vi "Link Channel.vi"(8 "error in (no error)":errorcluster, 11 "CIF_UI in":refnum<class "CIF_UI.lvclass">) -> (0 "error out":errorcluster, 3 "CIF_UI out":refnum<class "CIF_UI.lvclass">)   [LabVIEW 2021, in "CIF_UI.lvclass"]
uses:
  CIF_UI.lvclass
  CIF_UI.lvclass/CIF_UI.ctl
  CIFCore/Grpc/CIFCoreWrapper/CIFCoreWrapper.lvlib
  CIFCore/Grpc/CIFCoreChannel_client/RPC Messages/cif_channelcore_ConnectSubscriber.ctl
  CIFCore/Grpc/CIFCoreChannel_client/CIFCoreChannel_client.lvlib
  CIFCore/Common/CIFCoreCommon.lvlib
  CIFCore/Common/Typedef/Errors.ctl
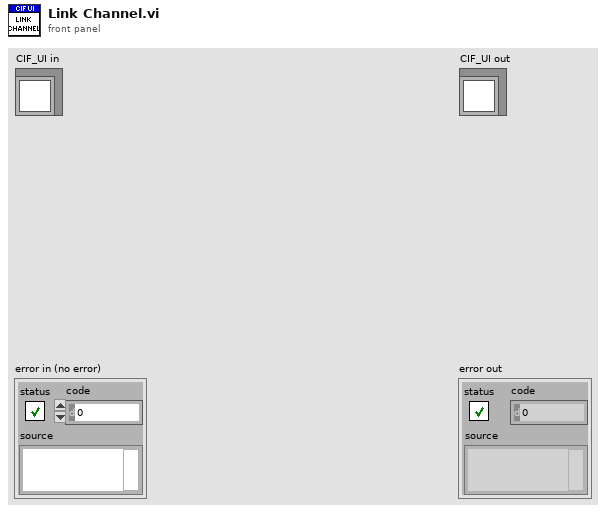
[diagram p1: front panel]
types:
  T1 = typedef "CIF_UI.lvclass/Plugin Connection Map.ctl" = map{string, T2}
  T2 = typedef "CIF_UI.lvclass/Plugin Connections.ctl" = cluster{"gRPC ID":T3, "Plugin info":T4}
  T3 = typedef "grpc-lvsupport-release.lvlib/grpcId.ctl" = u64
  T4 = typedef "CIF_Manager_client.lvlib/cif_manager_PluginInfo.ctl" = cluster{"plugin_name":string, "plugin_type":string, "grpc_port":i32, "plugin_version":T5, "status":T6}
  T5 = typedef "CIF_Manager_client.lvlib/cif_manager_PluginVersion.ctl" = cluster{"major_version":i32, "minor_version":i32, "fix_version":i32, "build_version":i32}
  T6 = typedef "CIF_Manager_client.lvlib/cif_plugincore_StatusData.ctl" = cluster{"state":T7, "timing_statistics":T8, "fifo_statistics":T10, "error":T11, "monitor_doubles":T12, "monitor_u64s":T13, "monitor_i64s":T14}
  T7 = typedef "CIF_Manager_client.lvlib/cif_plugincore_StatusData_State.ctl" = enum32{"NULL", "CREATING", "LISTENING", "RUNNING", "CLEANINGUP", "DESTROYING"}
  T8 = typedef "CIF_Manager_client.lvlib/cif_plugincore_TimingStatistics.ctl" = cluster{"period":T9, "wake_error":T9, "execute":T9, "housekeep":T9, "idle":T9}
  T9 = typedef "CIF_Manager_client.lvlib/cif_plugincore_TimingStatsBasic.ctl" = cluster{"max":i32, "min":i32}
  T10 = typedef "CIF_Manager_client.lvlib/cif_plugincore_FifoStatistics.ctl" = cluster{"from_t0":T9, "from_previous_plugin":T9, "output_error":T9}
  T11 = typedef "CIF_Manager_client.lvlib/cif_plugincore_Error.ctl" = cluster{"status":bool, "code":i32}
  T12 = typedef "CIF_Manager_client.lvlib/cif_plugincore_MonitorDoubles.ctl" = cluster{"double_1":dbl, "double_2":dbl, "double_3":dbl, "double_4":dbl}
  T13 = typedef "CIF_Manager_client.lvlib/cif_plugincore_MonitorU64.ctl" = cluster{"u64_1":u64, "u64_2":u64, "u64_3":u64, "u64_4":u64}
  T14 = typedef "CIF_Manager_client.lvlib/cif_plugincore_MonitorI64.ctl" = cluster{"i64_1":i64, "i64_2":i64, "i64_3":i64, "i64_4":i64}
  T15 = typedef "CIFCoreChannel_client.lvlib/cif_channelcore_ConnectSubscriber.ctl" = cluster{"subscriber_name":string, "publisher_name":string, "custom_connect":u8[]}
  T16 = typedef "CIFCoreCommon.lvlib/Errors.ctl" = enum16{"Invalid Clock ID", "Long Sleep", "gRPC Server Not Found", "Config Parse", "Timestamp Wrap", "Delayed Execution", "Duplicate Channel", "Missing Channel", "Incorrect Type", "Flatten Error", "Unflatten Data", "Unique Name", "Plugin Not Found", "Plugin Type Not Found", "Plugin Version Not Found", "Manager Not Found", "Numerical Issue", "Time Jump", "Clock ID Match", "Channel Length", "Plugin Connection"}
  T17 = typedef "CIF_UI.lvclass/Channel Connection.ctl" = cluster{"Subscriber Name":string, "Publisher Name":string, "Custom Data":string}
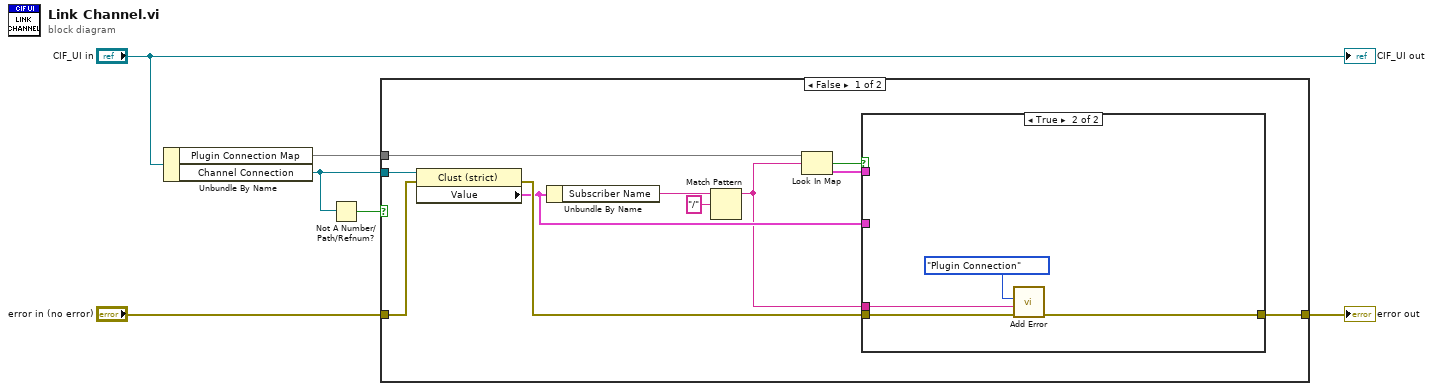
[diagram p0: block diagram]
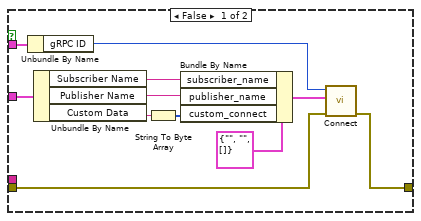
[diagram p2: hidden frame]
diagram:
  n1 = Unbundle By Name("CIF_UI in") -> ("Plugin Connection Map"=w4:T1, "Channel Connection"=w2:refnum<vi>)
  n2 = Not A Number/Path/Refnum?(number/path/refnum=w2) -> (NaN/Path/Refnum?=w1:bool)
  n3 = case shown="False" w1 {
    tunnel: "error in (no error)" -> [w17 w33]
    tunnel: w4 -> [w12 _]
    tunnel: [w9 w33] -> w3
    tunnel: w2 -> [w8 _]
    frame False {
      n4 = property class="Clust (strict)"(reference=w8, error in=w17) -> (error out=w14:errorcluster, "Value"=w13:T17)  [unwired: 1 out]
      n5 = Unbundle By Name(w13) -> ("Subscriber Name"=w16:string)
      n6 = Match Pattern(string=w16, regular expression="/") -> (before substring=w7:string)  [unwired: 1 in, 3 out]
      n7 = Look In Map(map=w12, key=w7) -> (key not found?=w11:bool, value=w10:T2)  [unwired: 1 in]
      n8 = case shown="True" w11 {
        tunnel: w14 -> [w19 w32]
        tunnel: w10 -> [w28 _]
        tunnel: w13 -> [w20 _]
        tunnel: [w18 w31] -> w9
        tunnel: w7 -> [_ w30]
        frame False {
          n9 = Unbundle By Name(w28) -> ("gRPC ID"=w21:T3)
          n10 = Unbundle By Name(w20) -> ("Subscriber Name"=w27:string, "Publisher Name"=w26:string, "Custom Data"=w24:string)
          n11 = String To Byte Array(string=w24) -> (unsigned byte array=w25:u8[])
          n12 = Bundle By Name(cluster=T15 {"subscriber_name"="", "publisher_name"="", "custom_connect"=[]} ("Connection 2"), "subscriber_name"=w27, "publisher_name"=w26, "custom_connect"=w25) -> (w22:T15)
          n13 = call "Connect.vi"("error in"=w19, "Connection"=w22, "gRPC ID"=w21) -> ("error out"=w18:errorcluster)  [unwired: 7 in, 1 out]
        }
        frame True {
          n14 = call "Add Error.vi"("error in (no error)"=w32, "String to Append"=w30, "Error"=Errors."Plugin Connection") -> ("error out"=w31:errorcluster)  [unwired: 8 in]
        }
      }
    }
    frame True {
    }
  }
  "error out" <- w3
  "CIF_UI out" <- "CIF_UI in"
